vi "Set Flow Control.vi"(8 "error in (no error)":errorcluster, 11 "Handle":u32) -> (0 "error out":errorcluster, 2 "COM port":string, 3 "Handle out":u32)   [LabVIEW 2019, in "D2XX-lv.lvlib"]
uses:
  D2XX-lv.lvlib
  D2XX_Functions_7.0/D2XX.lvlib
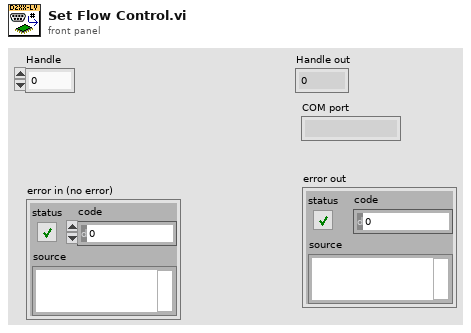
[diagram p1: front panel]
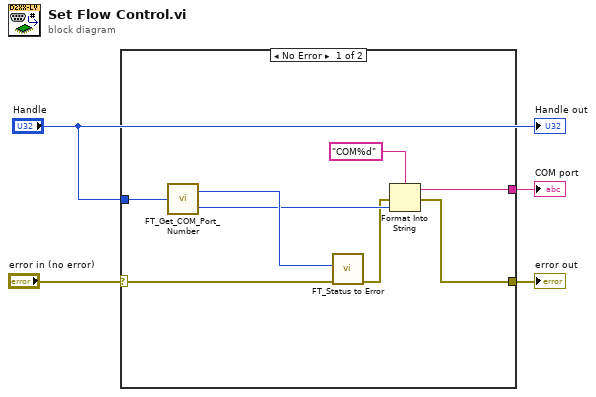
[diagram p0: block diagram]
diagram:
  n1 = case shown="No Error" "error in (no error)" {
    selector: "error in (no error)" -> [w12 w13]
    tunnel: [w6 w13] -> w3
    tunnel: "Handle" -> [w11 _]
    tunnel: [w5 _] -> w1
    frame No Error {
      n2 = call "FT_Get_COM_Port_Number.vi"("Handle"=w11) -> ("FT_Status"=w10:u32, "COM Port Number"=w8:i32)
      n3 = call "FT_Status to Error.vi"("error in (no error)"=w12, "FT_Status"=w10) -> ("error out"=w7:errorcluster)  [unwired: 9 in]
      n4 = Format Into String(format string="COM%d", error in=w7, w8) -> (resulting string=w5:string, error out=w6:errorcluster)  [unwired: 1 in]
    }
    frame Error {
    }
  }
  "error out" <- w3
  "COM port" <- w1
  "Handle out" <- "Handle"
